vi "运维调试.vi"() -> ()   [LabVIEW 2016]
uses:
  <vilib>/Utility/miscctls.llb/LVPointTypeDef.ctl
  PLC/PLC.lvlib
  <vilib>/Utility/config.llb/NI_LVConfig.lvlib
panel:
  in  "运维调试菜单":T1(xcontrol)
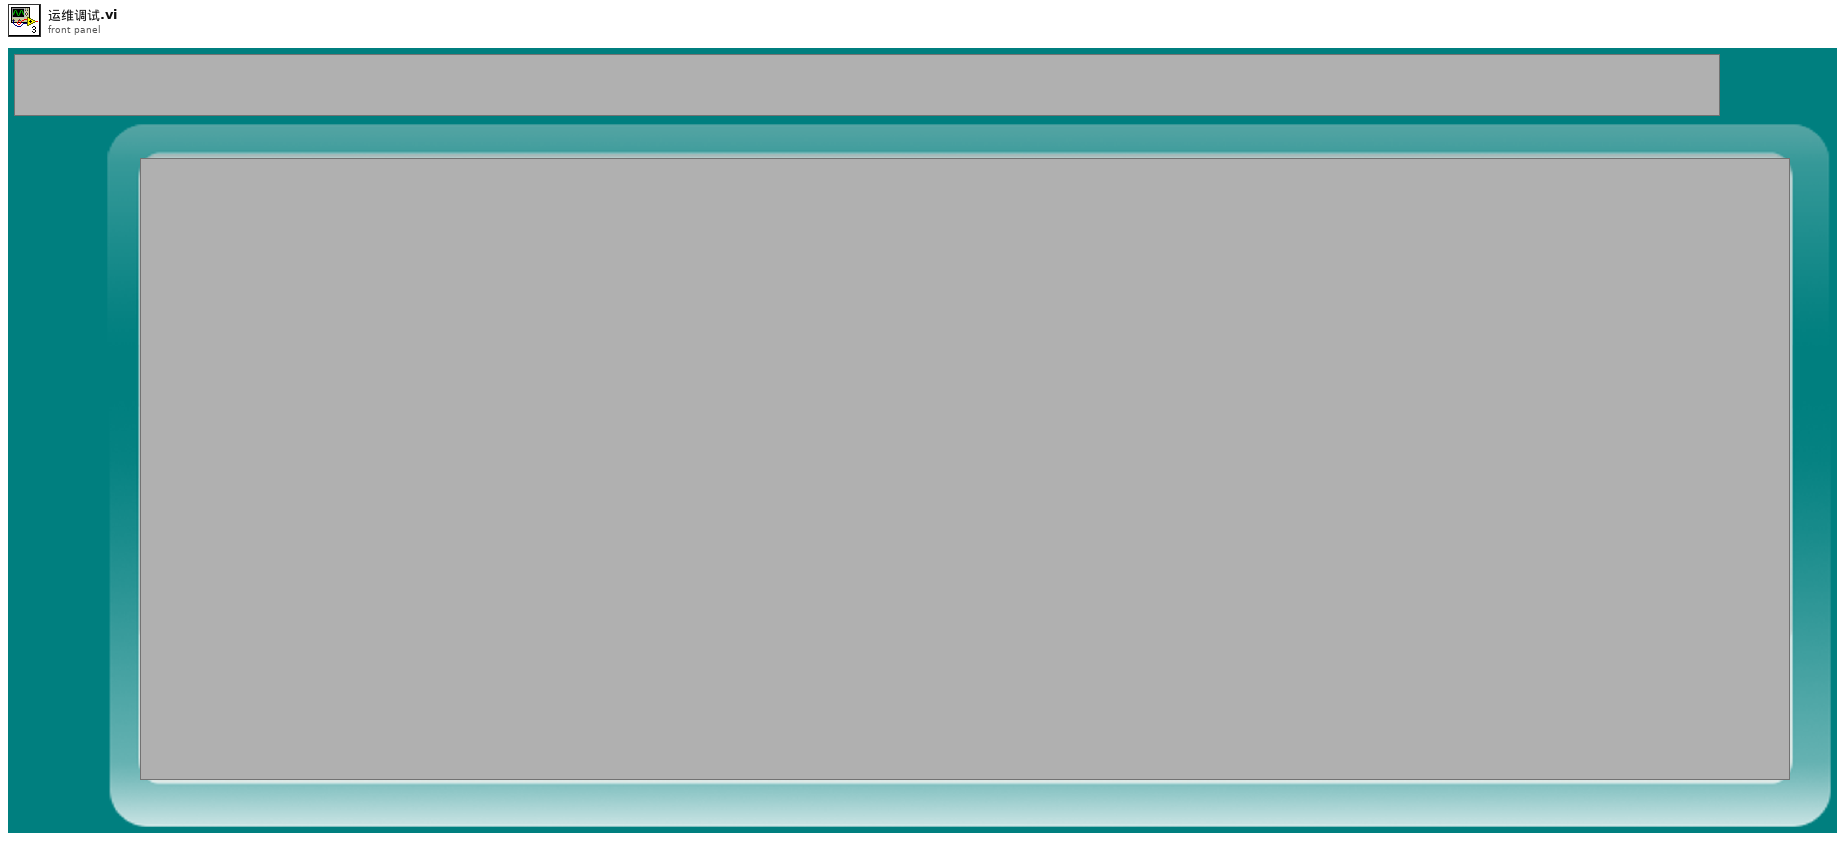
[diagram p1: front panel]
types:
  T1 = enum16{"电源管理", "采配水", "氨氮", "总磷总氮", "多参数", "CODMn", "CODcr", "流量计", "质控单元", "超标留样", "其他"}
  T2 = typedef "NI_LVConfig.lvlib/Config Data RefNum.ctl" = refnum<k1>
  T3 = typedef "LVPointTypeDef.ctl" = cluster{"Horizontal":i16, "Vertical":i16}
  T4 = enum16{"Enabled", "Disabled", "Disabled and Grayed Out"}
  T5 = enum32{"Bad", "Idle", "Run top level", "Running"}
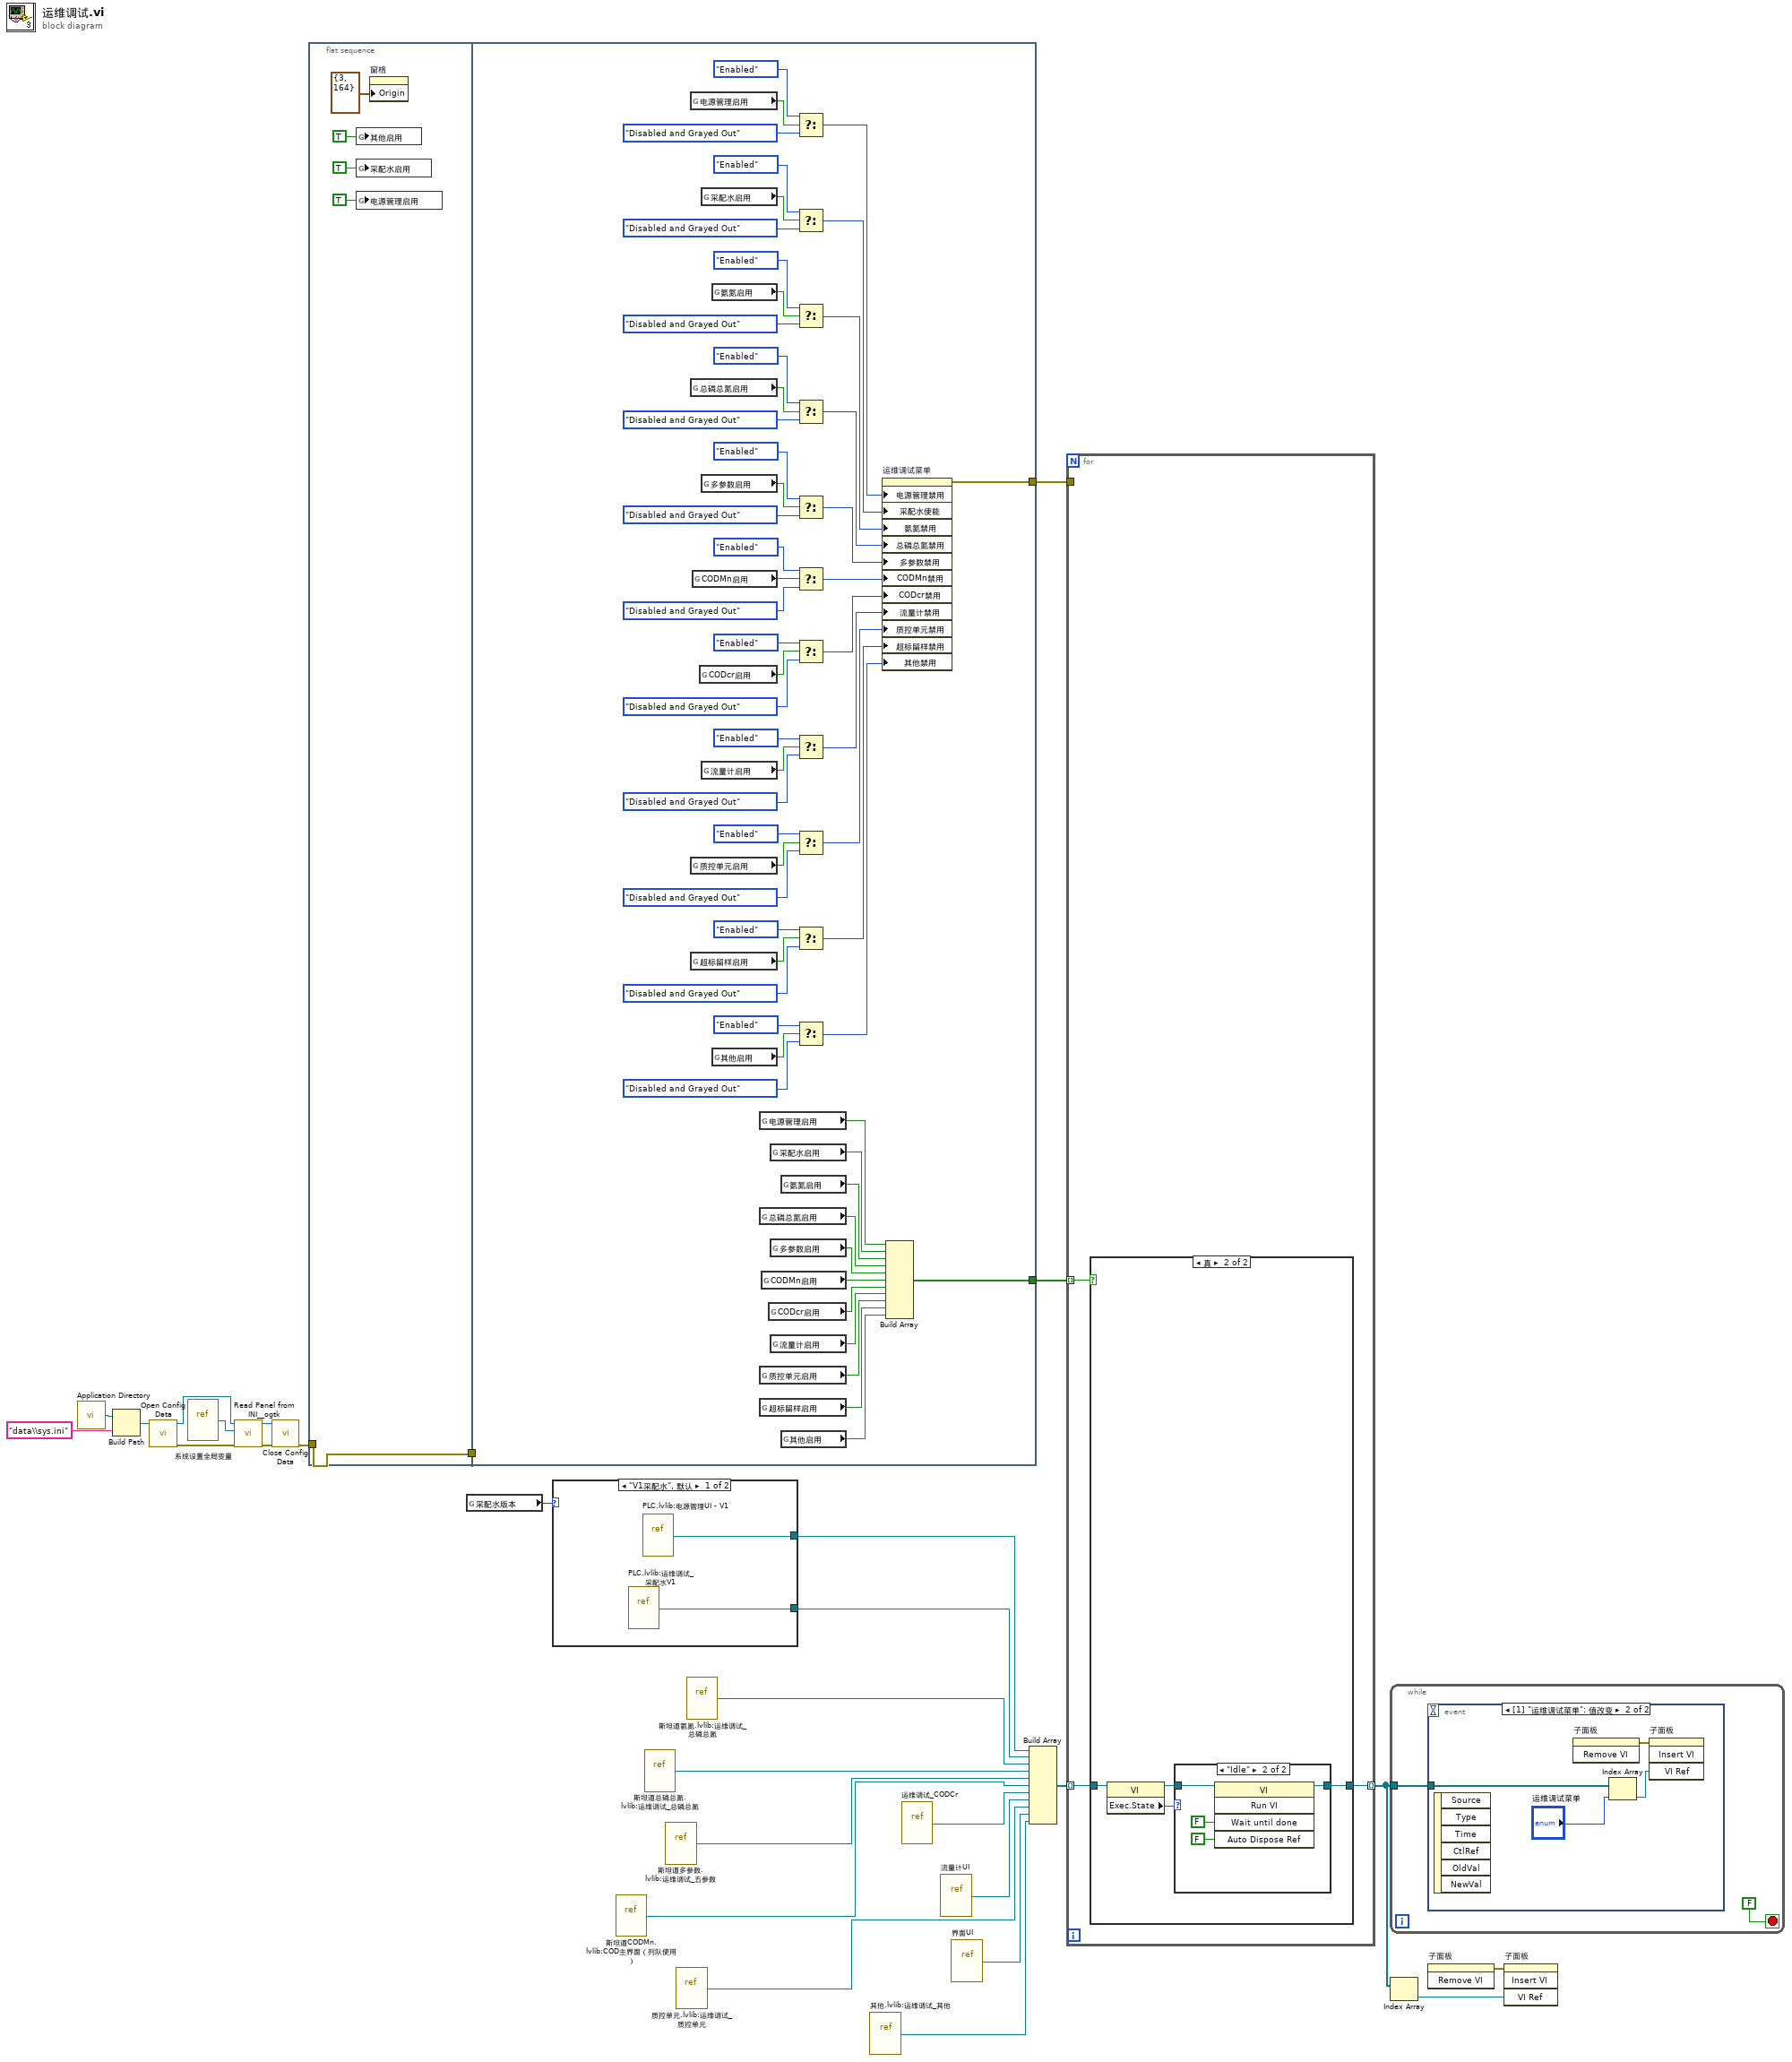
[diagram p0: block diagram]
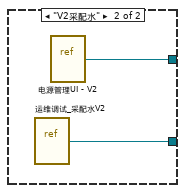
[diagram p2: hidden frame]
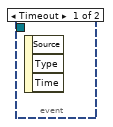
[diagram p5: hidden frame]
diagram:
  n1 = call <vilib>:"Application Directory.vi"() -> ("Application Directory"=w8:path)
  n2 = Build Path(base path=w8, name or relative path="data\\sys.ini" ("名称或相对路径")) -> (appended path=w6:path)
  n3 = call <vilib>:"Open Config Data.vi"("configuration file path"=w6) -> ("error out"=w15:errorcluster, "refnum"=w14:T2)  [unwired: 8 in, 1 out]
  n4 = vi-ref "系统设置全局变量.vi"() -> (w13:refnum<vi>)
  n5 = call <userlib>:"Read Panel from INI__ogtk.vi"("error in (no error)"=w15, "VI ref"=w13, "refnum"=w14) -> ("error out"=w12:errorcluster, "refnum out"=w11:T2)  [unwired: 7 in]
  n6 = call <vilib>:"Close Config Data.vi"("error in (no error)"=w12, "refnum"=w11) -> ("error out"=w10:errorcluster)  [unwired: 8 in, 1 out]
  n7 = flat-sequence {
    tunnel: w10 -> [w33]
    tunnel: [w33] -> w9
    tunnel: [w71] -> w16
    tunnel: w9 -> [_]
    tunnel: [w61] -> w5
    frame #0 {
      n8 = global write "系统设置全局变量.vi" "其他启用"(TRUE ("其他启用")) -> ()
      n9 = global write "系统设置全局变量.vi" "采配水启用"(TRUE ("采配水启用")) -> ()
      n10 = global write "系统设置全局变量.vi" "电源管理启用"(TRUE ("电源管理启用")) -> ()
      n11 = property on="窗格" class="Pane"("Origin"=T3 {"Horizontal"=3, "Vertical"=164} ("原点")) -> ()  [unwired: 2 in, 2 out]
    }
    frame #1 {
      n12 = global read "系统设置全局变量.vi" "电源管理启用"() -> (w90:bool)
      n13 = global read "系统设置全局变量.vi" "总磷总氮启用"() -> (w84:bool)
      n14 = global read "系统设置全局变量.vi" "质控单元启用"() -> (w77:bool)
      n15 = global read "系统设置全局变量.vi" "超标留样启用"() -> (w35:bool)
      n16 = global read "系统设置全局变量.vi" "CODMn启用"() -> (w80:bool)
      n17 = global read "系统设置全局变量.vi" "CODcr启用"() -> (w79:bool)
      n18 = global read "系统设置全局变量.vi" "采配水启用"() -> (w87:bool)
      n19 = global read "系统设置全局变量.vi" "多参数启用"() -> (w82:bool)
      n20 = global read "系统设置全局变量.vi" "流量计启用"() -> (w78:bool)
      n21 = global read "系统设置全局变量.vi" "氨氮启用"() -> (w86:bool)
      n22 = global read "系统设置全局变量.vi" "其他启用"() -> (w76:bool)
      n23 = global read "系统设置全局变量.vi" "电源管理启用"() -> (w62:bool)
      n24 = global read "系统设置全局变量.vi" "总磷总氮启用"() -> (w65:bool)
      n25 = global read "系统设置全局变量.vi" "质控单元启用"() -> (w70:bool)
      n26 = global read "系统设置全局变量.vi" "超标留样启用"() -> (w40:bool)
      n27 = global read "系统设置全局变量.vi" "CODMn启用"() -> (w67:bool)
      n28 = global read "系统设置全局变量.vi" "CODcr启用"() -> (w68:bool)
      n29 = global read "系统设置全局变量.vi" "采配水启用"() -> (w63:bool)
      n30 = global read "系统设置全局变量.vi" "多参数启用"() -> (w66:bool)
      n31 = global read "系统设置全局变量.vi" "流量计启用"() -> (w69:bool)
      n32 = global read "系统设置全局变量.vi" "氨氮启用"() -> (w64:bool)
      n33 = global read "系统设置全局变量.vi" "其他启用"() -> (w39:bool)
      n34 = Select(t=T4."Enabled" ("电源管理禁用"), s=w90, f=T4."Disabled and Grayed Out" ("电源管理禁用")) -> (s? t:f=w89:T4)
      n35 = Select(t=T4."Enabled" ("电源管理禁用"), s=w87, f=T4."Disabled and Grayed Out" ("电源管理禁用")) -> (s? t:f=w88:T4)
      n36 = Select(t=T4."Enabled" ("电源管理禁用"), s=w86, f=T4."Disabled and Grayed Out" ("电源管理禁用")) -> (s? t:f=w85:T4)
      n37 = Select(t=T4."Enabled" ("电源管理禁用"), s=w84, f=T4."Disabled and Grayed Out" ("电源管理禁用")) -> (s? t:f=w83:T4)
      n38 = Select(t=T4."Enabled" ("电源管理禁用"), s=w82, f=T4."Disabled and Grayed Out" ("电源管理禁用")) -> (s? t:f=w81:T4)
      n39 = Select(t=T4."Enabled" ("电源管理禁用"), s=w80, f=T4."Disabled and Grayed Out" ("电源管理禁用")) -> (s? t:f=w75:T4)
      n40 = Select(t=T4."Enabled" ("电源管理禁用"), s=w79, f=T4."Disabled and Grayed Out" ("电源管理禁用")) -> (s? t:f=w74:T4)
      n41 = Select(t=T4."Enabled" ("电源管理禁用"), s=w78, f=T4."Disabled and Grayed Out" ("电源管理禁用")) -> (s? t:f=w73:T4)
      n42 = Select(t=T4."Enabled" ("电源管理禁用"), s=w77, f=T4."Disabled and Grayed Out" ("电源管理禁用")) -> (s? t:f=w72:T4)
      n43 = Select(t=T4."Enabled" ("电源管理禁用"), s=w35, f=T4."Disabled and Grayed Out" ("电源管理禁用")) -> (s? t:f=w34:T4)
      n44 = Select(t=T4."Enabled" ("电源管理禁用"), s=w76, f=T4."Disabled and Grayed Out" ("电源管理禁用")) -> (s? t:f=w38:T4)
      n45 = property on="运维调试菜单" class="运维调试菜单 (严格)"("电源管理禁用"=w89, "采配水使能"=w88, "氨氮禁用"=w85, "总磷总氮禁用"=w83, "多参数禁用"=w81, "CODMn禁用"=w75, "CODcr禁用"=w74, "流量计禁用"=w73, "质控单元禁用"=w72, "超标留样禁用"=w34, "其他禁用"=w38) -> (error out=w71:errorcluster)  [unwired: 2 in, 1 out]
      n46 = Build Array(w62, w63, w64, w65, w66, w67, w68, w69, w70, w40, w39) -> (w61:bool[])
    }
  }
  n47 = global read "系统设置全局变量.vi" "采配水版本"() -> (w2:enum16{"V1采配水", "V2采配水"})
  n48 = case shown="\"V1采配水\", 默认" w2 {
    tunnel: [w92 w94] -> w18
    tunnel: [w91 w93] -> w1
    frame "V1采配水", Default {
      n49 = vi-ref "PLC.lvlib:运维调试_采配水V1.vi"() -> (w91:refnum<vi>)
      n50 = vi-ref "PLC.lvlib:电源管理UI - V1.vi"() -> (w92:refnum<vi>)
    }
    frame "V2采配水" {
      n51 = vi-ref "运维调试_采配水V2.vi"() -> (w93:refnum<vi>)
      n52 = vi-ref "电源管理UI - V2.vi"() -> (w94:refnum<vi>)
    }
  }
  n53 = vi-ref "斯坦道CODMn.lvlib:COD主界面（列队使用）.vi"() -> (w21:refnum<vi>)
  n54 = vi-ref "斯坦道总磷总氮.lvlib:运维调试_总磷总氮.vi"() -> (w23:refnum<vi>)
  n55 = vi-ref "斯坦道多参数.lvlib:运维调试_五参数.vi"() -> (w22:refnum<vi>)
  n56 = vi-ref "质控单元.lvlib:运维调试_质控单元.vi"() -> (w19:refnum<vi>)
  n57 = vi-ref "斯坦道氨氮.lvlib:运维调试_总磷总氮.vi"() -> (w24:refnum<vi>)
  n58 = vi-ref "其他.lvlib:运维调试_其他.vi"() -> (w3:refnum<vi>)
  n59 = vi-ref "运维调试_CODCr.vi"() -> (w20:refnum<vi>)
  n60 = vi-ref "流量计UI.vi"() -> (w17:refnum<vi>)
  n61 = vi-ref "界面UI.vi"() -> (w4:refnum<vi>)
  n62 = Build Array(w18, w1, w24, w23, w22, w21, w20, w17, w19, w4, w3) -> (w25:refnum<vi>[])
  n63 = for {
    tunnel: w25 -> [w97] mode=indexing
    tunnel: [w96] -> w27 mode=indexing
    tunnel: w5 -> [w95] mode=indexing
    tunnel: w16 -> [_]
    n64 = case shown="真" w95 {
      tunnel: w97 -> [w98 w102]
      tunnel: [w98 w99] -> w96
      frame False {
      }
      frame True {
        n65 = property class="VI"(reference=w102) -> (reference out=w100:refnum<vi>, "Exec.State"=w101:T5)  [unwired: 1 in, 1 out]
        n66 = case shown="\"Idle\"" w101 {
          tunnel: w100 -> [w103 w105]
          tunnel: [w103 w104] -> w99
          frame "Bad", Default {
          }
          frame "Idle" {
            n67 = invoke class="VI" method="Run VI"(reference=w105, "Wait until done"=FALSE ("结束前等待"), "Auto Dispose Ref"=FALSE ("自动销毁引用")) -> (reference out=w104:refnum<vi>)  [unwired: 2 in, 4 out]
          }
        }
      }
    }
  }
  n68 = while {
    tunnel: w27 -> [w108]
    stop <- FALSE stop-if-true
    n69 = event shown="[1] \"运维调试菜单\": 值改变" {
      selector: _ -> [_ _]
      dyn-events: _ -> [_ _]
      timeout: _ -> [_ _]
      tunnel: w108 -> [_ w112]
      event Timeout {
        n70 = event-data() -> ()  [unwired: 1 in, 3 out]
      }
      event "运维调试菜单": Value Change {
        n71 = event-data() -> ()  [unwired: 1 in, 6 out]
        n72 = invoke on="子面板" class="SubPnl" method="Remove VI"() -> (error out=w113:errorcluster)  [unwired: 3 in, 2 out]
        n73 = Index Array(array=w112, index="运维调试菜单") -> (element=w111:refnum<vi>)
        n74 = invoke on="子面板" class="SubPnl" method="Insert VI"(error in=w113, "VI Ref"=w111) -> ()  [unwired: 2 in, 4 out]
      }
    }
  }
  n75 = Index Array(array=w27) -> (element=w26:refnum<vi>)  [unwired: 1 in]
  n76 = invoke on="子面板" class="SubPnl" method="Remove VI"() -> (error out=w28:errorcluster)  [unwired: 3 in, 2 out]
  n77 = invoke on="子面板" class="SubPnl" method="Insert VI"(error in=w28, "VI Ref"=w26) -> ()  [unwired: 2 in, 4 out]
